vi "Actor Core.vi"(8 "error in":errorcluster, 11 "hydraharp_panel in":refnum<class "hydraharp_panel.lvclass">) -> (0 "error out":errorcluster, 3 "Actor out":refnum<class "Actor.lvclass">)   [LabVIEW 2015, in "hydraharp_panel.lvclass"]
doc: "(<B>Filename</B>: Actor Framework.lvlib:Actor.lvclass:Actor Core.vi)\n\nReceives messages to the actor, reacts to them, and initiates any error handling that may shut the actor down.\n\nDescendant classes may override this VI to append parallel tasks for the actor to complete while it handles messages. Overrides use the Call Parent Method node."
uses:
  hydraharp_panel.lvclass
  <vilib>/ActorFramework/Actor/Actor.lvclass
  hpanel_hydraharp_settings.ctl
  hpanel_sync_settings.ctl
  hpanel_sync_div.ctl
  hpanel_channel_settings.ctl
  hpanel_acq_modes.ctl
  hpanel_hydrharp_tasks.ctl
  hydraharp/hydraharp_correlation_lag_settings.ctl
  hydraharp/hydraharp_time_decades.ctl
  hpanel_control_references.ctl
  UI/panel_class/panel.lvclass/panel.ctl
  <vilib>/ActorFramework/Actor/Actor.lvclass/Actor.ctl
  <vilib>/ActorFramework/Message Enqueuer/Message Enqueuer.lvclass/Message Enqueuer.ctl
  hydraharp_panel.lvclass/hydraharp_panel.ctl
  hydraharp_panel Messages/connect_to_hydraharp Msg/connect_to_hydraharp Msg.lvclass/connect_to_hydraharp Msg.ctl
  record_type.ctl
  hydraharp/hydraharp_action_on_records.ctl
  hydraharp_panel Messages/stream_TTTR Msg/stream_TTTR Msg.lvclass/stream_TTTR Msg.ctl
  hpanel_correlation_settings.ctl
  hydraharp_panel Messages/change_hydraharp_settings Msg/change_hydraharp_settings Msg.lvclass/change_hydraharp_settings Msg.ctl
  <vilib>/ActorFramework/Message Enqueuer/Init from Existing Queue.vi
  <vilib>/ActorFramework/Message Enqueuer/Enqueue.vi
  <vilib>/ActorFramework/Message Priority Queue/Priority Enqueue.vi
  <vilib>/ActorFramework/Message Enqueuer/Message Enqueuer.lvclass
  hydraharp_panel Messages/disconnect_from_hydraharp Msg/disconnect_from_hydraharp Msg.lvclass
  hydraharp_panel Messages/connect_to_hydraharp Msg/connect_to_hydraharp Msg.lvclass
  hydraharp_panel Messages/get_current_count_rates Msg/get_current_count_rates Msg.lvclass
  hydraharp_panel Messages/stream_TTTR Msg/stream_TTTR Msg.lvclass
  hydraharp_panel Messages/change_hydraharp_settings Msg/change_hydraharp_settings Msg.lvclass
  UI/panel_class/panel.lvclass
panel:
  in  "save_settings":bool
  out "error out 2":errorcluster
  in  "stop_task":bool
  in  "do_task":bool
  in  "Task":T1
  in  "chart_channels":bool
  in  "Mode":T2=2 items=["T2"=2, "T3"=3]
  out "Status":string
  in  "connect_hydraharp":bool
  in  "hydra_tab":enum32{"Basic Settings", "Advanced"}(tab)
  in  "Hydraharp Settings":T3={"Sync Settings"={"snc_count"=0, "snc_level"=50, "snc_ZeroX"=10, "snc_offs"=0, "sync_div"=enum."1"}, "CH 1"={"ch_counts"=0, "ch_level"=50, "ch_ZeroX"=10, "ch_offs"=0}, "CH 2"={"ch_counts"=0, "ch_level"=50, "ch_ZeroX"=10, "ch_offs"=0}, "CH 3"={"ch_counts"=0, "ch_level"=50, "ch_ZeroX"=10, "ch_offs"=0}, "CH 4"={"ch_counts"=0, "ch_level"=50, "ch_ZeroX"=10, "ch_offs"=0}, "binning"=1, "CH 5"={"ch_counts"=0, "ch_level"=0, "ch_ZeroX"=0, "ch_offs"=0}, "CH 6"={"ch_counts"=0, "ch_level"=0, "ch_ZeroX"=0, "ch_offs"=0}, "CH 7"={"ch_counts"=0, "ch_level"=0, "ch_ZeroX"=0, "ch_offs"=0}, "CH 8"={"ch_counts"=0, "ch_level"=0, "ch_ZeroX"=0, "ch_offs"=0}} {"CH 8"."ch_offs" min=-99999 max=99999 step=1; "CH 8"."ch_ZeroX" min=0 max=20 step=1; "CH 8"."ch_level" min=0 max=800 step=1; "CH 7"."ch_offs" min=-99999 max=99999 step=1; "CH 7"."ch_ZeroX" min=0 max=20 step=1; "CH 7"."ch_level" min=0 max=800 step=1; "CH 6"."ch_offs" min=-99999 max=99999 step=1; "CH 6"."ch_ZeroX" min=0 max=20 step=1; "CH 6"."ch_level" min=0 max=800 step=1; "CH 5"."ch_offs" min=-99999 max=99999 step=1; "CH 5"."ch_ZeroX" min=0 max=20 step=1; "CH 5"."ch_level" min=0 max=800 step=1; "binning" min=0 max=10 step=1; "CH 4"."ch_offs" min=-99999 max=99999 step=1; "CH 4"."ch_ZeroX" min=0 max=20 step=1; "CH 4"."ch_level" min=0 max=800 step=1; "CH 3"."ch_offs" min=-99999 max=99999 step=1; "CH 3"."ch_ZeroX" min=0 max=20 step=1; "CH 3"."ch_level" min=0 max=800 step=1; "CH 2"."ch_offs" min=-99999 max=99999 step=1; "CH 2"."ch_ZeroX" min=0 max=20 step=1; "CH 2"."ch_level" min=0 max=800 step=1; "CH 1"."ch_offs" min=-99999 max=99999 step=1; "CH 1"."ch_ZeroX" min=0 max=20 step=1; "CH 1"."ch_level" min=0 max=800 step=1; "Sync Settings"."snc_offs" min=-99999 max=99999 step=1; "Sync Settings"."snc_ZeroX" min=0 max=20 step=1; "Sync Settings"."snc_level" min=0 max=800 step=10}
  in  "Stream Notes":string
  in  "acq_time (s)":u32=1000
  in  "Stream Path":path
  in  "Ch2":u8 max=16
  in  "Ch1":u8 max=16
  in  "Lag Settings":T7={"time_start"=1000000, "time_end"=100000000000, "coarseness"=4} {"time_start" items=["1 ps"=1, "10 ps"=10, "100 ps"=100, "1 ns"=1000, "10 ns"=10000, "100 ns"=100000, "1 us"=1000000, "10 us"=10000000, "100 us"=100000000, "1 ms"=1000000000, "10 ms"=10000000000, "100 ms"=100000000000, "1 s"=1000000000000, "10 s"=10000000000000, "100 s"=100000000000000]; "time_end" items=["1 ps"=1, "10 ps"=10, "100 ps"=100, "1 ns"=1000, "10 ns"=10000, "100 ns"=100000, "1 us"=1000000, "10 us"=10000000, "100 us"=100000000, "1 ms"=1000000000, "10 ms"=10000000000, "100 ms"=100000000000, "1 s"=1000000000000, "10 s"=10000000000000, "100 s"=100000000000000]}
  in  "Save Records?":bool
  # "HydraHarp"
  # "Stream Settings"
  # "Correlation Settings"
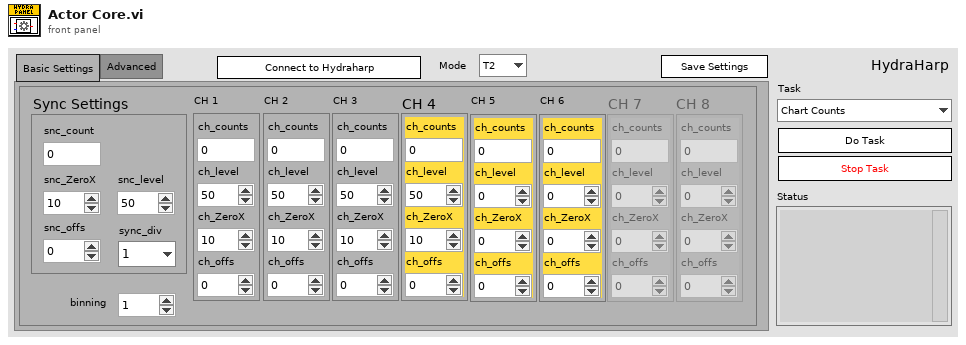
[diagram p1: front panel]
types:
  T1 = typedef "hpanel_hydrharp_tasks.ctl" = enum16{"Chart Counts", "Stream to File", "Plot Correlation", "Histogram"}
  T2 = typedef "hpanel_acq_modes.ctl" = u16
  T3 = typedef "hpanel_hydraharp_settings.ctl" = cluster{"Sync Settings":T4, "CH 1":T6, "CH 2":T6, "CH 3":T6, "CH 4":T6, "binning":i32, "CH 5":T6, "CH 6":T6, "CH 7":T6, "CH 8":T6}
  T4 = typedef "hpanel_sync_settings.ctl" = cluster{"snc_count":i32, "snc_level":i32, "snc_ZeroX":i32, "snc_offs":i32, "sync_div":T5}
  T5 = typedef "hpanel_sync_div.ctl" = enum16{"1", "2", "4", "8"}
  T6 = typedef "hpanel_channel_settings.ctl" = cluster{"ch_counts":i32, "ch_level":i32, "ch_ZeroX":i32, "ch_offs":i32}
  T7 = typedef "hydraharp_correlation_lag_settings.ctl" = cluster{"time_start":T8, "time_end":T8, "coarseness":i64}
  T8 = typedef "hydraharp_time_decades.ctl" = i64
  T9 = typedef "hpanel_control_references.ctl" = cluster{"Status":refnum<vi>, "snc_count":refnum<vi>, "ch1_counts":refnum<vi>, "ch2_counts":refnum<vi>, "ch3_counts":refnum<vi>, "ch4_counts":refnum<vi>, "ch5_counts":refnum<vi>, "ch6_counts":refnum<vi>, "ch7_counts":refnum<vi>, "ch8_counts":refnum<vi>}
  T10 = typedef "hpanel_user_events.ctl" = cluster{"message_panel":refnum<event-registration>, "stop_fifo_stream":refnum<event-registration>, "harp_status":refnum<event-registration>}
  T11 = cluster{"message_panel":refnum<event-registration>, "stop_ui_ref":refnum<event-registration>, "harp_status":refnum<event-registration>}
  T12 = enum16{"open", "replace", "create", "open or create", "replace or create", "replace or create with confirmation"}
  T13 = typedef "record_type.ctl" = enum16{"Raw Stream", "Processed Records (hdf5)"}
  T14 = enum8{"Enabled", "Disabled", "Disabled and Grayed Out"}
  T15 = typedef "hydraharp_action_on_records.ctl" = enum16{"stream_to_file", "correlate", "stream to file and correlate", "histogram"}
  T16 = typedef "hpanel_correlation_settings.ctl" = cluster{"Lag Settings":T7, "Ch1":u8, "Ch2":u8}
  T17 = typedef "ui_user_events.ctl" = cluster{"update_xy_graph":refnum<user-event>, "update_graph":refnum<user-event>, "update_chart":refnum<user-event>, "update_map":refnum<user-event>, "event_loop_stop":refnum<user-event>, "keep_map":refnum<user-event>}
  T18 = typedef "messages_to_panel_from_actor_loop.ctl" = enum16{"reenable_tasks"}
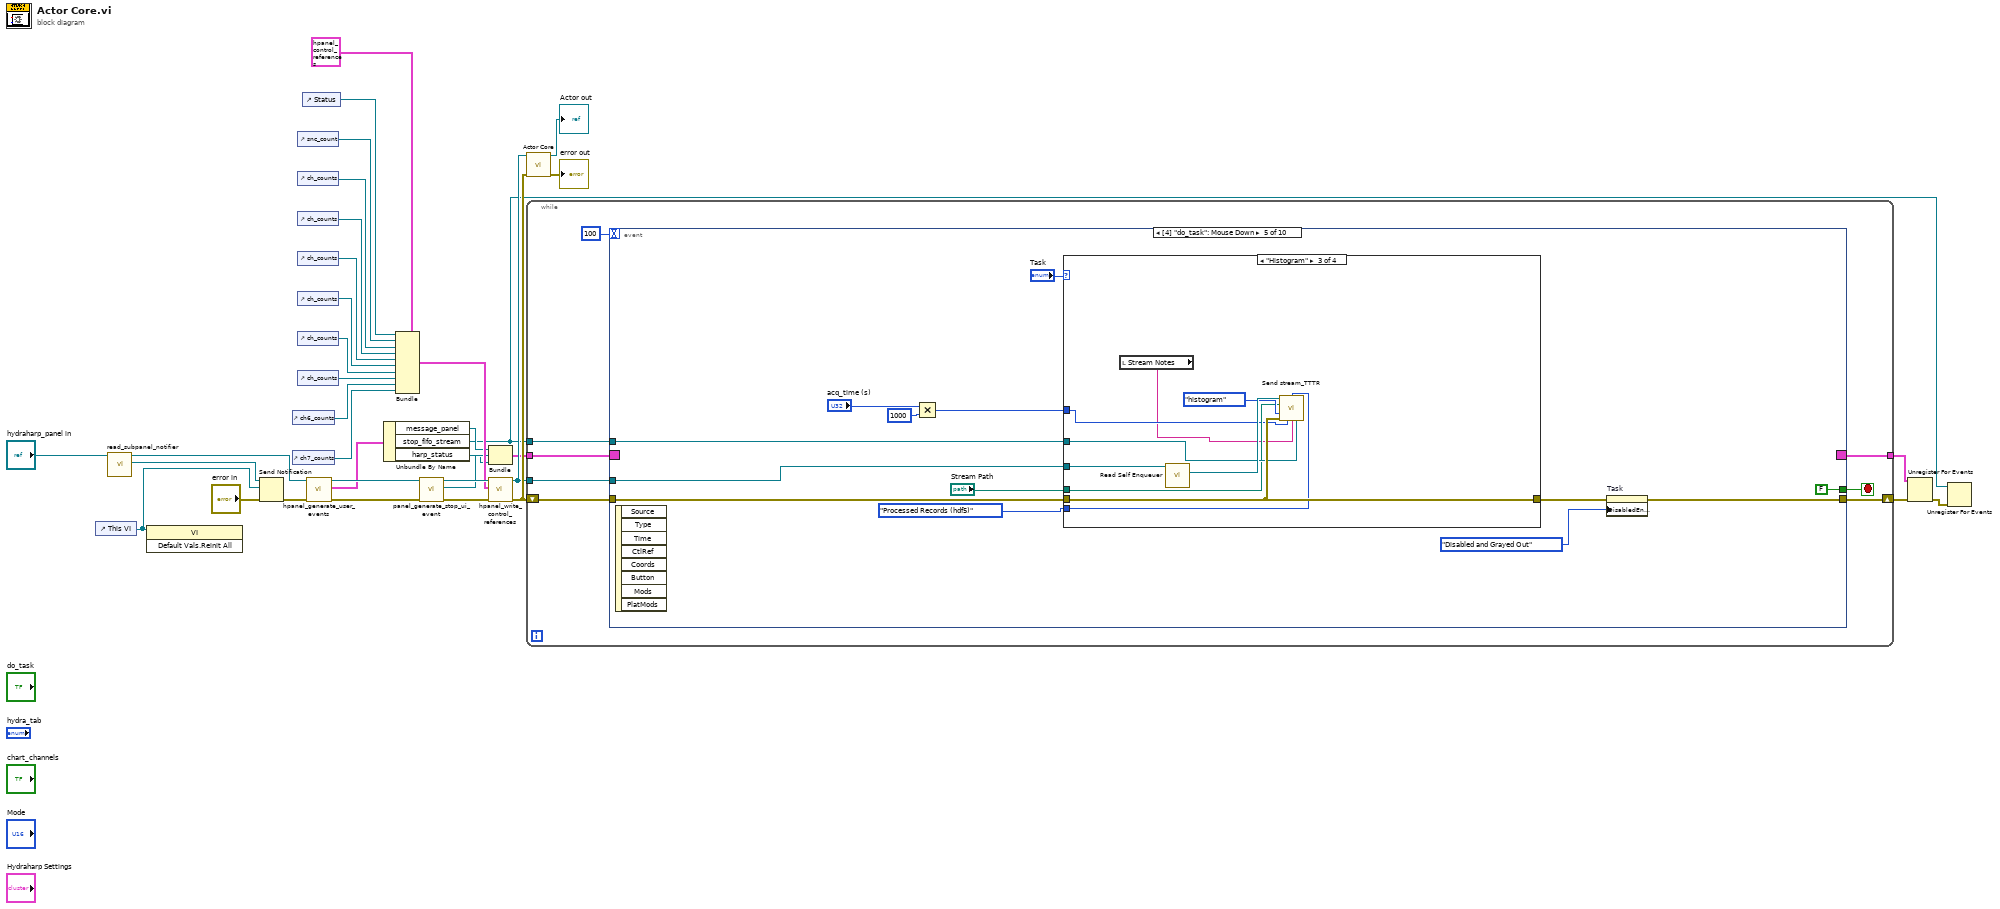
[diagram p0: block diagram]
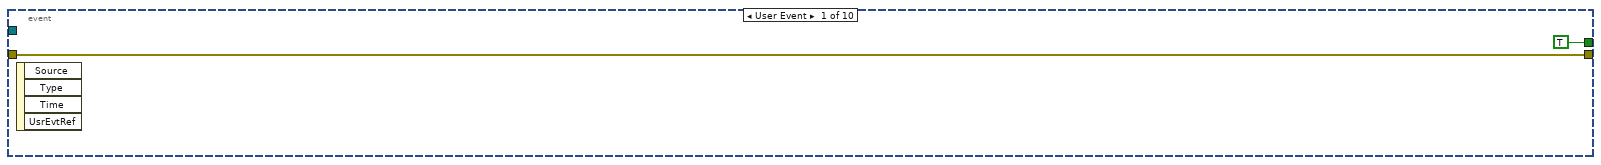
[diagram p2: hidden frame]
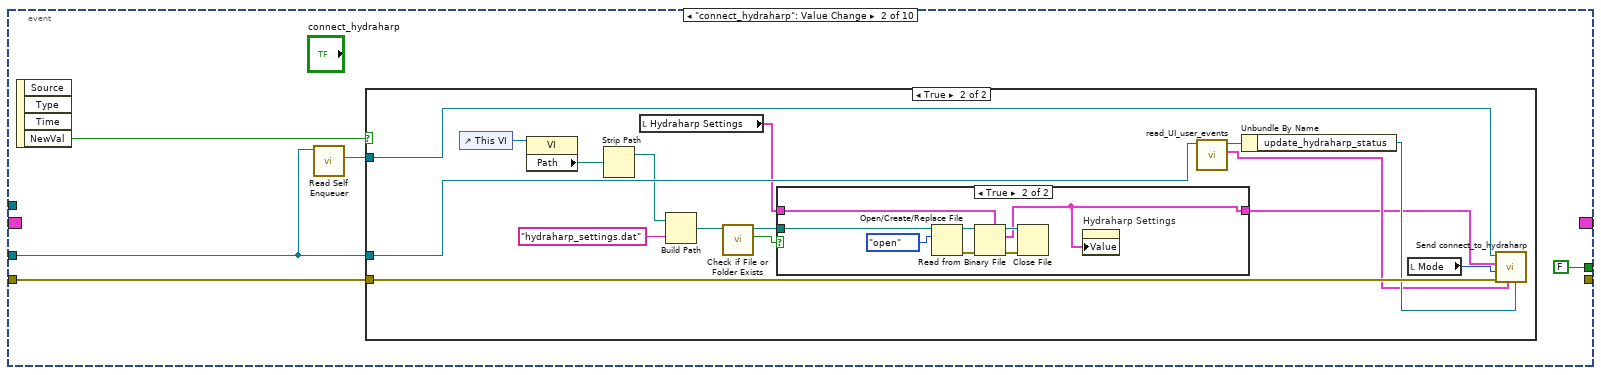
[diagram p3: hidden frame]
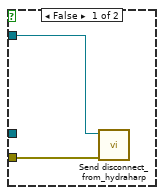
[diagram p4: hidden frame]
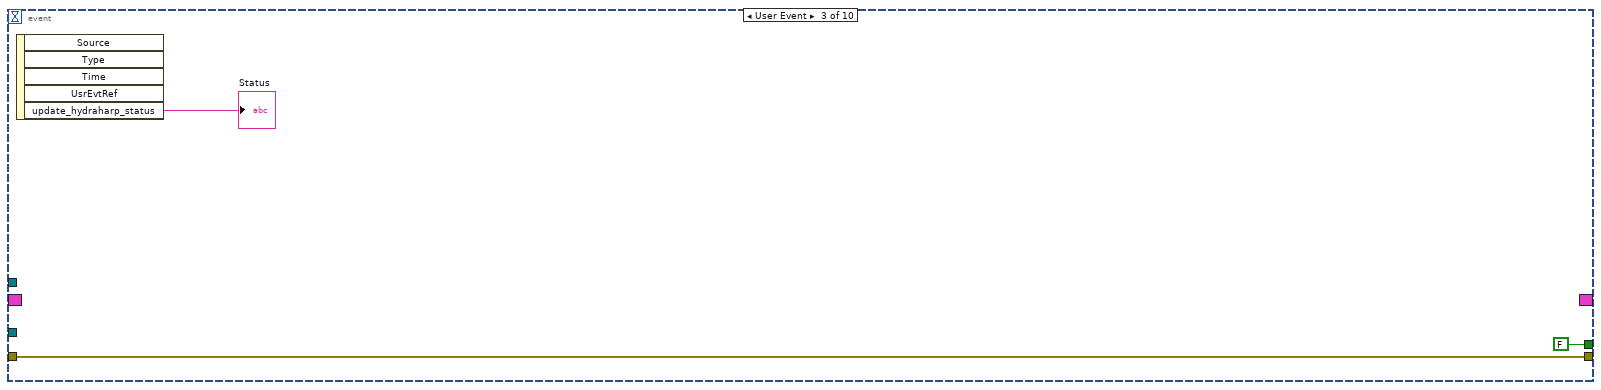
[diagram p6: hidden frame]
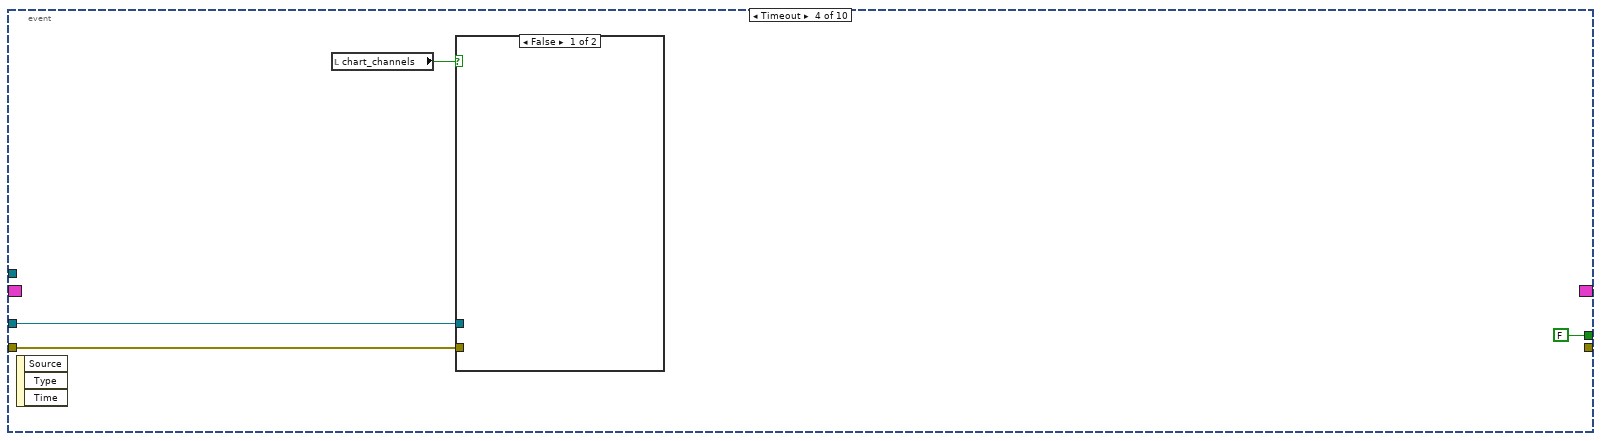
[diagram p7: hidden frame]
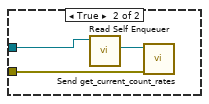
[diagram p8: hidden frame]
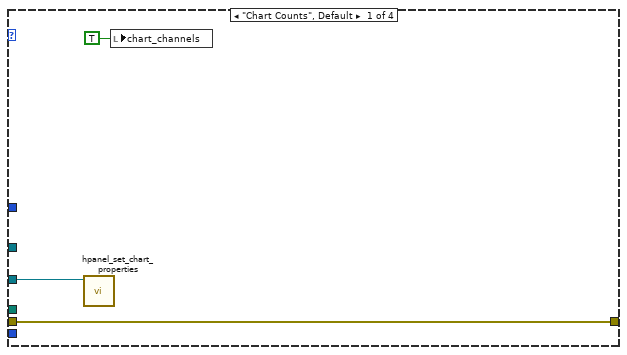
[diagram p9: hidden frame]
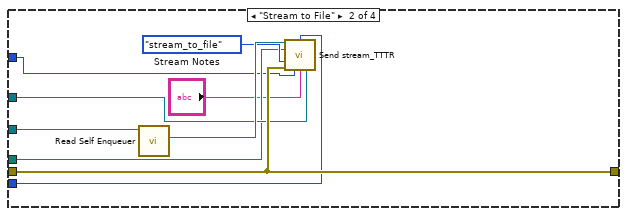
[diagram p10: hidden frame]
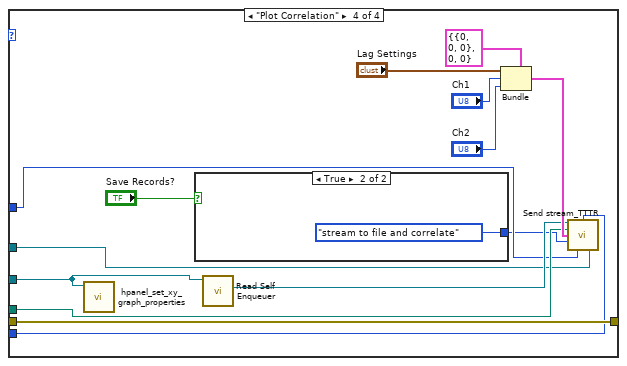
[diagram p11: hidden frame]
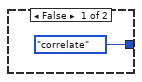
[diagram p12: hidden frame]
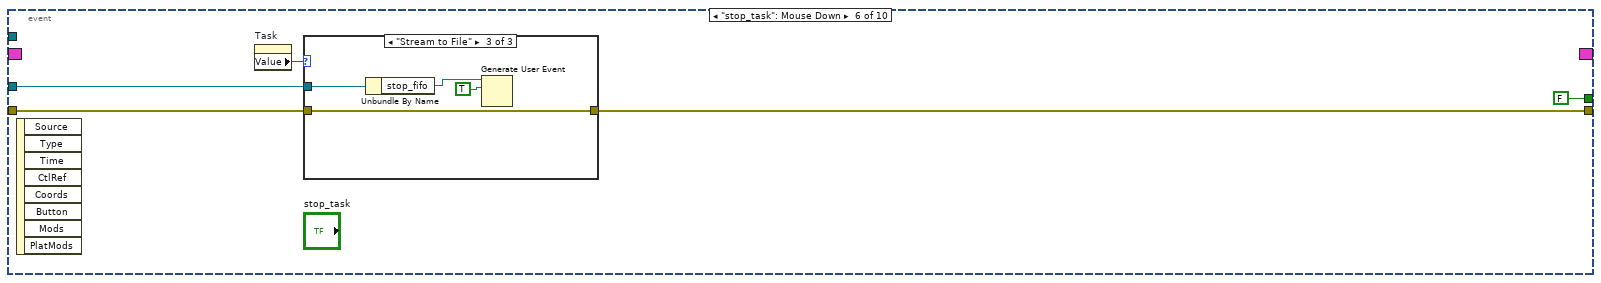
[diagram p13: hidden frame]
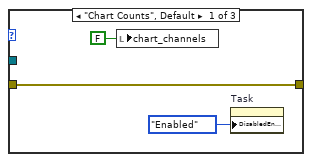
[diagram p14: hidden frame]
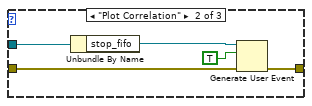
[diagram p15: hidden frame]
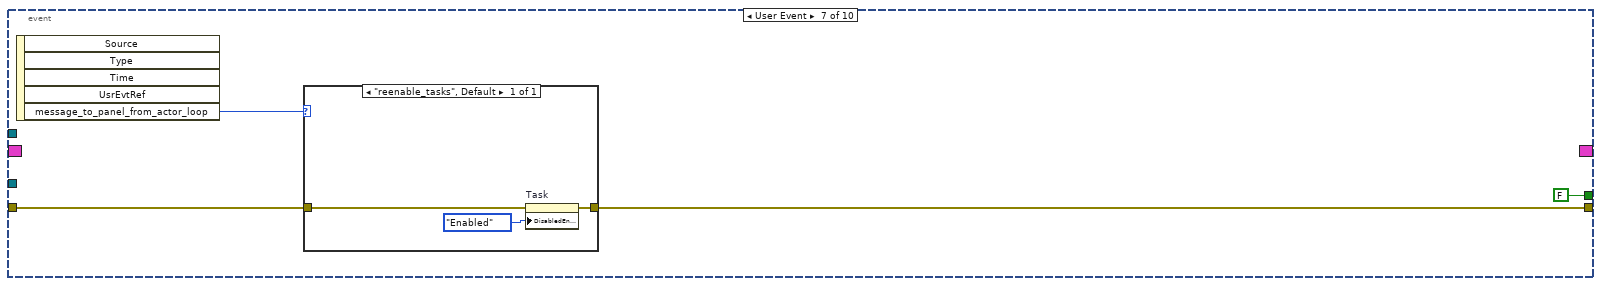
[diagram p16: hidden frame]
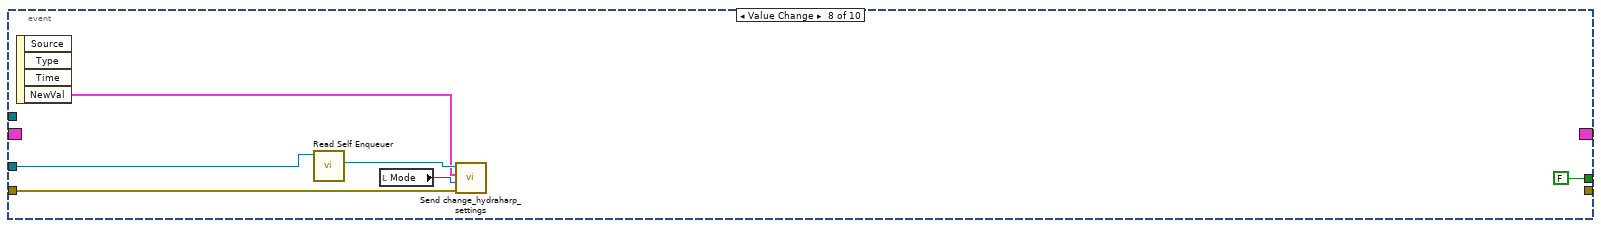
[diagram p17: hidden frame]
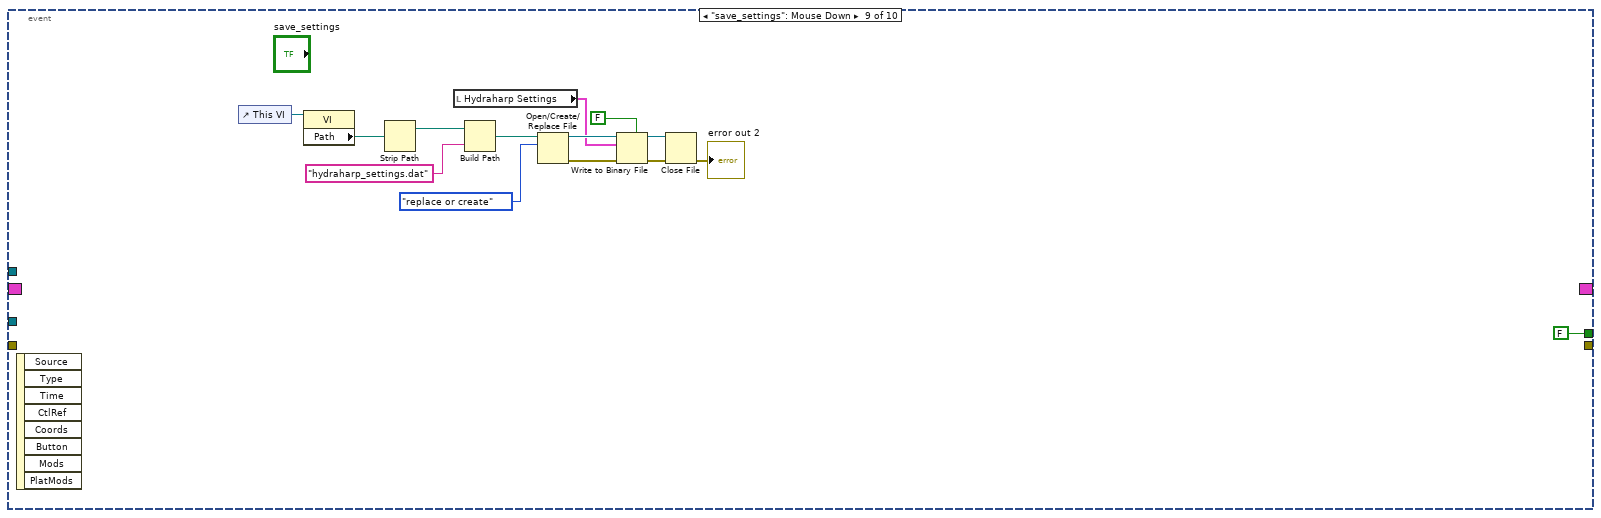
[diagram p18: hidden frame]
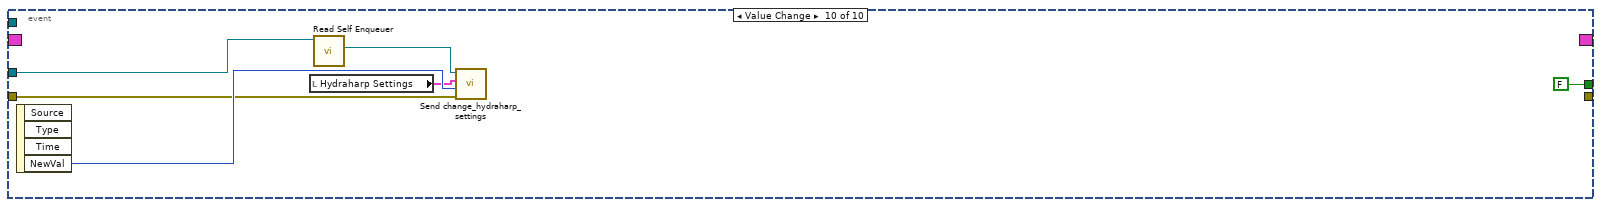
[diagram p19: hidden frame]
diagram:
  n1 = control-ref of="This VI"() -> (w18:refnum<vi>)
  n2 = call "read_subpanel_notifier.vi"("panel in"="hydraharp_panel in") -> ("subpanel_notifier"=w7:refnum<notifier>, "panel out"=w8:refnum<class "hydraharp_panel.lvclass">)  [unwired: 8 in, 1 out]
  n3 = invoke class="VI" method="Default Vals.Reinit All"(reference=w18) -> ()  [unwired: 2 in, 3 out]
  n4 = Send Notification(notification=w18, notifier=w7, error in (no error)="error in") -> (error out=w17:errorcluster)  [unwired: 1 out]
  n5 = control-ref of="ch6_counts"() -> (w6:refnum<vi>)
  n6 = control-ref of="ch7_counts"() -> (w5:refnum<vi>)
  n7 = control-ref of="snc_count"() -> (w29:refnum<vi>)
  n8 = control-ref of="ch_counts"() -> (w28:refnum<vi>)
  n9 = control-ref of="ch_counts"() -> (w27:refnum<vi>)
  n10 = control-ref of="ch_counts"() -> (w26:refnum<vi>)
  n11 = control-ref of="ch_counts"() -> (w25:refnum<vi>)
  n12 = control-ref of="ch_counts"() -> (w4:refnum<vi>)
  n13 = control-ref of="ch_counts"() -> (w3:refnum<vi>)
  n14 = control-ref of="Status"() -> (w30:refnum<vi>)
  n15 = call "hpanel_generate_user_events.vi"("error in (no error)"=w17, "hydraharp_panel in"=w8) -> ("error out"=w16:errorcluster, "events"=w13:T10, "hydraharp_panel out"=w15:refnum<class "hydraharp_panel.lvclass">)  [unwired: 7 in]
  n16 = Unbundle By Name(w13) -> ("message_panel"=w12:refnum<event-registration>, "stop_fifo_stream"=w2:refnum<event-registration>, "harp_status"=w10:refnum<event-registration>)
  n17 = Bundle(cluster=T9 {"Status"=refnum, "snc_count"=refnum, "ch1_counts"=refnum, "ch2_counts"=refnum, "ch3_counts"=refnum, "ch4_counts"=refnum, "ch5_counts"=refnum, "ch6_counts"=refnum, "ch7_counts"=refnum, "ch8_counts"=refnum} ("output cluster"), "Status"=w30, "snc_count"=w29, "ch1_counts"=w28, "ch2_counts"=w27, "ch3_counts"=w26, "ch4_counts"=w25, "ch5_counts"=w4, "ch6_counts"=w3, "ch7_counts"=w6, "ch8_counts"=w5) -> (w20:T9)
  n18 = call "panel_generate_stop_ui_event.vi"("error in (no error)"=w16, "panel in"=w15) -> ("error out"=w22:errorcluster, "stop_ui_ref"=w14:refnum<event-registration>, "panel out"=w23:refnum<class "hydraharp_panel.lvclass">)  [unwired: 7 in]
  n19 = Bundle("message_panel"=w12, "stop_ui_ref"=w14, "harp_status"=w10) -> (w11:T11)  [unwired: 1 in]
  n20 = call "hpanel_write_control_references.vi"("error in (no error)"=w22, "references"=w20, "hydraharp_panel in"=w23) -> ("error out"=w21:errorcluster, "hydraharp_panel out"=w19:refnum<class "hydraharp_panel.lvclass">)  [unwired: 7 in]
  n21 = call-parent "Actor Core.vi"("error in"=w21, "Actor in"=w19) -> ("error out"=→"error out":errorcluster, "Actor out"=→"Actor out":refnum<class "Actor.lvclass">)  [unwired: 8 in]
  n22 = while {
    tunnel: [w43] -> w32
    shift-right: [w40] -> w31
    shift-left: w21 -> [w41]
    tunnel: w19 -> [w39]
    tunnel: w11 -> [w37]
    tunnel: w2 -> [w36]
    stop <- w42 stop-if-true
    n23 = event shown="[4] \"do_task\": Mouse Down" {
      selector: w37 -> [_ _ _ _ _ _ _ _ _ _]
      dyn-events: [_ _ _ _ _ _ _ _ _ _] -> w43
      timeout: 100 -> [_ _ _ _ _ _ _ _ _ _]
      tunnel: [TRUE FALSE FALSE FALSE FALSE FALSE FALSE FALSE FALSE FALSE] -> w42
      tunnel: w41 -> [w44 w50 w78 w82 w98 w141 w156 w163 _ w183]
      tunnel: [w44 _ w78 _ w96 w138 w155 _ _ _] -> w40
      tunnel: w39 -> [_ w46 _ w83 w94 w139 _ w167 _ w187]
      tunnel: w36 -> [_ _ _ _ w93 _ _ _ _ _]
      event User Event {
        n24 = event-data() -> ()  [unwired: 1 in, 4 out]
      }
      event "connect_hydraharp": Value Change {
        n25 = event-data() -> ("NewVal"=w48:bool)  [unwired: 1 in, 3 out]
        n26 = call <vilib>:"Read Self Enqueuer.vi"("Actor"=w46) -> ("Self Enqueuer"=w49:refnum<class "Message Enqueuer.lvclass">)  [unwired: 10 in]
        n27 = case shown="True" w48 {
          tunnel: w50 -> [w51 w68]
          tunnel: w49 -> [w52 w67]
          tunnel: w46 -> [_ w64]
          frame False {
            n28 = call "Send disconnect_from_hydraharp.vi"("error in (no error)"=w51, "Message Enqueuer"=w52) -> ()  [unwired: 8 in, 2 out]
          }
          frame True {
            n29 = control-ref of="This VI"() -> (w61:refnum<vi>)
            n30 = property class="VI"(reference=w61) -> ("Path"=w60:path)  [unwired: 1 in, 2 out]
            n31 = Strip Path(path=w60) -> (stripped path=w59:path)  [unwired: 1 out]
            n32 = local read "Hydraharp Settings"() -> (w54:T3)
            n33 = Build Path(base path=w59, name or relative path="hydraharp_settings.dat") -> (appended path=w57:path)
            n34 = call <vilib>:"Check if File or Folder Exists.vi"("path"=w57) -> ("file or folder exists?"=w56:bool, "dup path"=w55:path)  [unwired: 8 in, 1 out]
            n35 = case shown="True" w56 {
              tunnel: w55 -> [_ w76]
              tunnel: w54 -> [w69 w73]
              tunnel: [w69 w70] -> w53
              frame False {
              }
              frame True {
                n36 = Open/Create/Replace File(file path (use dialog)=w76, operation (0:open)=T12."open") -> (refnum out=w75:refnum<file>, error out=w74:errorcluster)  [unwired: 4 in, 1 out]
                n37 = Read from Binary File(5:w73, 8:w74, 11:w75) -> (0:w72:errorcluster, 2:w70:T3, 3:w71:refnum<file>)  [unwired: 3 in, 1 out]
                n38 = Close File(refnum=w71, error in=w72) -> ()  [unwired: 2 out]
                n39 = property on="Hydraharp Settings" class="Clust (strict)"("Value"=w70) -> ()  [unwired: 2 in, 2 out]
              }
            }
            n40 = call "read_UI_user_events.vi"("panel in"=w64) -> ("ui_user_events"=w63:T17, "panel out"=w62:refnum<class "hydraharp_panel.lvclass">)  [unwired: 8 in, 1 out]
            n41 = Unbundle By Name(w62) -> ("update_hydraharp_status"=w65:refnum<user-event>)
            n42 = local read "Mode"() -> (w66:T2)
            n43 = call "Send connect_to_hydraharp.vi"("update_hydraharp_status"=w65, "ui_events"=w63, "error in (no error)"=w68, "Mode"=w66, "Hydraharp Settings"=w53, "Message Enqueuer"=w67) -> ()  [unwired: 4 in, 2 out]
          }
        }
      }
      event User Event {
        n44 = event-data() -> ("update_hydraharp_status"=→"Status":string)  [unwired: 1 in, 4 out]
      }
      event Timeout {
        n45 = event-data() -> ()  [unwired: 1 in, 3 out]
        n46 = local read "chart_channels"() -> (w81:bool)
        n47 = case shown="False" w81 {
          tunnel: w83 -> [_ w87]
          tunnel: w82 -> [_ w85]
          frame False {
          }
          frame True {
            n48 = call <vilib>:"Read Self Enqueuer.vi"("Actor"=w87) -> ("Self Enqueuer"=w86:refnum<class "Message Enqueuer.lvclass">)  [unwired: 10 in]
            n49 = call "Send get_current_count_rates.vi"("error in (no error)"=w85, "Message Enqueuer"=w86) -> ()  [unwired: 8 in, 2 out]
          }
        }
      }
      event "do_task": Mouse Down {
        n50 = event-data() -> ()  [unwired: 1 in, 8 out]
        n51 = Multiply(x="acq_time (s)", y=u32 1000) -> (x*y=w89:u32)
        n52 = case shown="\"Histogram\"" "Task" {
          tunnel: w98 -> [w103 w112 w121 w126]
          tunnel: [w103 w112 w121 w126] -> w97
          tunnel: w94 -> [w101 w106 w115 w124]
          tunnel: w93 -> [_ w109 w118 w123]
          tunnel: "Stream Path" -> [_ w108 w117 w129]
          tunnel: record_type."Processed Records (hdf5)" ("Record Type") -> [_ w105 w114 w122]
          tunnel: w89 -> [_ w107 w116 w128]
          frame "Chart Counts", Default {
            n53 = call "hpanel_set_chart_properties.vi"("hydraharp_panel in"=w101) -> ()  [unwired: 11 in]
            n54 = local write "chart_channels"(TRUE ("chart_channels")) -> ()
          }
          frame "Stream to File" {
            n55 = call <vilib>:"Read Self Enqueuer.vi"("Actor"=w106) -> ("Self Enqueuer"=w111:refnum<class "Message Enqueuer.lvclass">)  [unwired: 10 in]
            n56 = call "Send stream_TTTR.vi"("Message Enqueuer"=w111, "Log Type"=w105, "fifo_stream_path"=w108, "action_for_records"=hydraharp_action_on_records."stream_to_file", "error in (no error)"=w112, "acq_time"=w107, "Stream Notes"="Stream Notes", "stop_fifo_stream"=w109) -> ()  [unwired: 6 in, 2 out]
          }
          frame "Histogram" {
            n57 = local read "Stream Notes"() -> (w113:string)
            n58 = call <vilib>:"Read Self Enqueuer.vi"("Actor"=w115) -> ("Self Enqueuer"=w120:refnum<class "Message Enqueuer.lvclass">)  [unwired: 10 in]
            n59 = call "Send stream_TTTR.vi"("Message Enqueuer"=w120, "Log Type"=w114, "fifo_stream_path"=w117, "action_for_records"=hydraharp_action_on_records."histogram", "error in (no error)"=w121, "acq_time"=w116, "Stream Notes"=w113, "stop_fifo_stream"=w118) -> ()  [unwired: 6 in, 2 out]
          }
          frame "Plot Correlation" {
            n60 = call "hpanel_set_xy_graph_properties.vi"("hydraharp_panel in"=w124) -> ()  [unwired: 11 in]
            n61 = case shown="True" "Save Records?" {
              tunnel: [hydraharp_action_on_records."correlate" ("action_for_records") hydraharp_action_on_records."stream to file and correlate" ("action_for_records")] -> w127
              frame False {
              }
              frame True {
              }
            }
            n62 = call <vilib>:"Read Self Enqueuer.vi"("Actor"=w124) -> ("Self Enqueuer"=w130:refnum<class "Message Enqueuer.lvclass">)  [unwired: 10 in]
            n63 = Bundle(cluster=T16 {"Lag Settings"={"time_start"=0, "time_end"=0, "coarseness"=0}, "Ch1"=0, "Ch2"=0} ("output cluster"), "Lag Settings"="Lag Settings", "Ch1"="Ch1", "Ch2"="Ch2") -> (w131:T16)
            n64 = call "Send stream_TTTR.vi"("Message Enqueuer"=w130, "Log Type"=w122, "fifo_stream_path"=w129, "Correlation_settings"=w131, "action_for_records"=w127, "acq_time"=w128, "stop_fifo_stream"=w123) -> ()  [unwired: 7 in, 2 out]
          }
        }
        n65 = property on="Task" class="Enum (strict)"(error in=w97, "DisabledEnum"=T14."Disabled and Grayed Out" ("Disabled")) -> (error out=w96:errorcluster)  [unwired: 1 in, 1 out]
      }
      event "stop_task": Mouse Down {
        n66 = event-data() -> ()  [unwired: 1 in, 8 out]
        n67 = property on="Task" class="Enum (strict)"() -> ("Value"=w142:T1)  [unwired: 2 in, 2 out]
        n68 = case shown="\"Stream to File\"" w142 {
          tunnel: w141 -> [w144 w147 w153]
          tunnel: [w144 w146 w153] -> w138
          tunnel: w139 -> [_ w148 w152]
          frame "Chart Counts", Default {
            n69 = local write "chart_channels"(FALSE ("chart_channels")) -> ()
            n70 = property on="Task" class="Enum (strict)"("DisabledEnum"=T14."Enabled" ("Disabled")) -> ()  [unwired: 2 in, 2 out]
          }
          frame "Plot Correlation" {
            n71 = Unbundle By Name(w148) -> ("stop_fifo"=w149:refnum<user-event>)
            n72 = Generate User Event(user event=w149, event data cluster=TRUE ("event data"), error in=w147) -> (error out=w146:errorcluster)  [unwired: 1 in, 1 out]
          }
          frame "Stream to File" {
            n73 = Unbundle By Name(w152) -> ("stop_fifo"=w151:refnum<user-event>)
            n74 = Generate User Event(user event=w151, event data cluster=TRUE ("event data")) -> ()  [unwired: 2 in, 2 out]
          }
        }
      }
      event User Event {
        n75 = event-data() -> ("message_to_panel_from_actor_loop"=w158:T18)  [unwired: 1 in, 4 out]
        n76 = case shown="\"reenable_tasks\", Default" w158 {
          tunnel: w156 -> [w160]
          tunnel: [w159] -> w155
          frame "reenable_tasks", Default {
            n77 = property on="Task" class="Enum (strict)"(error in=w160, "DisabledEnum"=T14."Enabled" ("Disabled")) -> (error out=w159:errorcluster)  [unwired: 1 in, 1 out]
          }
        }
      }
      event Value Change {
        n78 = event-data() -> ("NewVal"=w162:T3)  [unwired: 1 in, 3 out]
        n79 = call <vilib>:"Read Self Enqueuer.vi"("Actor"=w167) -> ("Self Enqueuer"=w166:refnum<class "Message Enqueuer.lvclass">)  [unwired: 10 in]
        n80 = local read "Mode"() -> (w165:T2)
        n81 = call "Send change_hydraharp_settings.vi"("error in (no error)"=w163, "Mode"=w165, "Hydraharp Settings"=w162, "Message Enqueuer"=w166) -> ()  [unwired: 6 in, 2 out]
      }
      event "save_settings": Mouse Down {
        n82 = event-data() -> ()  [unwired: 1 in, 8 out]
        n83 = control-ref of="This VI"() -> (w181:refnum<vi>)
        n84 = property class="VI"(reference=w181) -> ("Path"=w180:path)  [unwired: 1 in, 2 out]
        n85 = Strip Path(path=w180) -> (stripped path=w179:path)  [unwired: 1 out]
        n86 = local read "Hydraharp Settings"() -> (w169:T3)
        n87 = Build Path(base path=w179, name or relative path="hydraharp_settings.dat") -> (appended path=w177:path)
        n88 = Open/Create/Replace File(file path (use dialog)=w177, operation (0:open)=T12."replace or create") -> (refnum out=w175:refnum<file>, error out=w174:errorcluster)  [unwired: 4 in, 1 out]
        n89 = Write to Binary File(file (use dialog)=w175, data=w169, error in=w174, 5:FALSE ("prepend array or string size? (T)")) -> (refnum out=w171:refnum<file>, error out=w172:errorcluster)  [unwired: 2 in, 1 out]
        n90 = Close File(refnum=w171, error in=w172) -> (error out=→"error out 2":errorcluster)  [unwired: 1 out]
      }
      event Value Change {
        n91 = event-data() -> ("NewVal"=w185:T2)  [unwired: 1 in, 3 out]
        n92 = local read "Hydraharp Settings"() -> (w184:T3)
        n93 = call <vilib>:"Read Self Enqueuer.vi"("Actor"=w187) -> ("Self Enqueuer"=w186:refnum<class "Message Enqueuer.lvclass">)  [unwired: 10 in]
        n94 = call "Send change_hydraharp_settings.vi"("error in (no error)"=w183, "Mode"=w185, "Hydraharp Settings"=w184, "Message Enqueuer"=w186) -> ()  [unwired: 6 in, 2 out]
      }
    }
  }
  n95 = Unregister For Events(event registration refnum=w32, error in=w31) -> (error out=w1:errorcluster)
  n96 = Unregister For Events(event registration refnum=w2, error in=w1) -> ()  [unwired: 1 out]
